vi "Close.vi"(8 "error in (no error)":errorcluster, 11 "Test Group Manager in":refnum<class "Test Group Manager.lvclass">) -> (0 "error out":errorcluster, 3 "Test Group Manager out":refnum<class "Test Group Manager.lvclass">)   [LabVIEW 2016, in "Test Group Manager.lvlib" / "Test Group Manager.lvclass"]
uses:
  Test Group Manager.lvclass
  Test Group Manager.lvclass/Test Group Manager.ctl
  Includes/Test Group/Test Group.lvclass
  Protected Methods/Read Test Group Database.vi
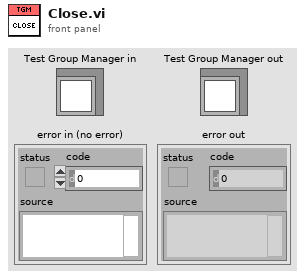
[diagram p1: front panel]
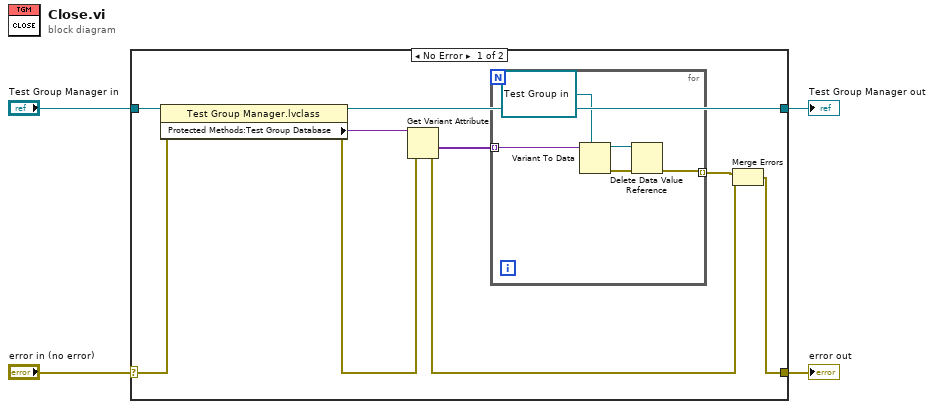
[diagram p0: block diagram]
diagram:
  n1 = case shown="No Error" "error in (no error)" {
    selector: "error in (no error)" -> [w13 w20]
    tunnel: [w5 w20] -> w3
    tunnel: [w11 w19] -> w1
    tunnel: "Test Group Manager in" -> [w12 w19]
    frame No Error {
      n2 = property class="Test Group Manager.lvclass"(reference=w12, error in=w13) -> (reference out=w11:refnum<class "Test Group Manager.lvclass">, error out=w9:errorcluster, "Protected Methods:Test Group Database"=w10:variant)
      n3 = Get Variant Attribute(Variant=w10, error in=w9) -> (values=w8:variant[], error out=w6:errorcluster)  [unwired: 2 in, 2 out]
      n4 = for {
        tunnel: w8 -> [w18] mode=indexing
        tunnel: [w14] -> w7 mode=indexing
        n5 = Variant To Data(type=refnum<data-value> refnum ("Test Group In"), Variant=w18) -> (data=w15:refnum<data-value>, error out=w16:errorcluster)  [unwired: 1 in]
        n6 = Delete Data Value Reference(data value reference=w15, error in=w16) -> (error out=w14:errorcluster)  [unwired: 1 out]
      }
      n7 = Merge Errors(w7, w6) -> (w5:errorcluster)
    }
    frame Error {
    }
  }
  "error out" <- w3
  "Test Group Manager out" <- w1
